vi "Main.vi"() -> ()   [LabVIEW 2011]
uses:
  2-Think/2 Typedefs/Which Boat.ctl
  2-Think/2 Typedefs/UTM Circle.ctl
  0x2-OCU-Think Comm/0x2 Typedefs/Waypoints List.ctl
  2-Think/2 Classes/Waypoint/Waypoint.lvclass
  0x2-OCU-Think Comm/0x2 Typedefs/Current Waypoint.ctl
  2-Think/2 Typedefs/eStopCommand.ctl
  0x2-OCU-Think Comm/0x2 Typedefs/ocuMessage.ctl
  0x2-OCU-Think Comm/0x2 Typedefs/ocuCommands.ctl
  <vilib>/Platform/TimedLoop/XDataNode/timing_clust.ctl
  <vilib>/Platform/TimedLoop/XDataNode/nitl_modes.ctl
  <vilib>/Platform/TimedLoop/XDataNode/wakeup.ctl
  <vilib>/vision/Image Controls.llb/IMAQ Image.ctl
  2-Think/2 Globals/2 Global.vi
  2-Think/2 Globals/2 Message Logger.vi
  <vilib>/Platform/TimedLoop/XDataNode/XDataNode.xnode
  <vilib>/Platform/TimedLoop/XDataNode/XDNodeRunTimeDep.lvlib
  0x2-OCU-Think Comm/0x2 Classes/NetworkStreams/Writer/NetworkStreamWriter.lvclass
  0x2-OCU-Think Comm/0x2 Classes/NetworkStreams/Reader/NetworkStreamReader.lvclass
  2-Think/2 Classes/Logger/Logger.lvclass
panel:
  in  "Skip Sense (->manual input only!)":bool
  in  "Enable logging?":bool=TRUE
  in  "Data storage folder":path
  in  "Which Boat Am I?\n(unnecessary to set on RIO)":T1=enum."Simulation"
  out "E-stop freq.":dbl
  out "Act freq.":dbl
  out "Sense freq.":dbl
  out "Think freq.":dbl
  in  "E-Stop":bool
  # "this is the parent VI under which \nSense Think and Act run."
  # "Will save to U:\\Logs when run on the RIO"
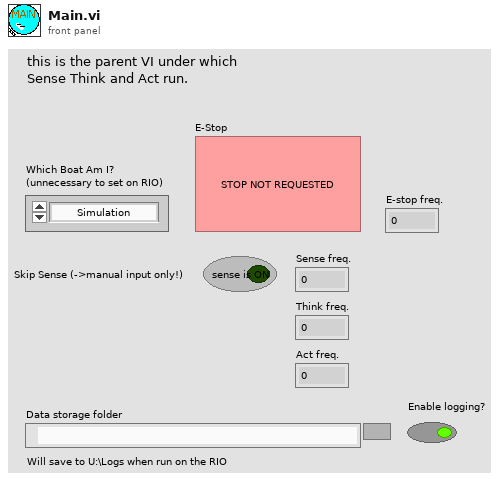
[diagram p1: front panel]
types:
  T1 = typedef "Which Boat.ctl" = enum16{"Competition Boat", "Small RC", "Simulation"}
  T2 = typedef "UTM Circle.ctl" = cluster{"UTM Zone":dbl, "Hemisphere":enum16{"North", "South"}, "East":dbl, "North":dbl, "Radius":dbl}
  T3 = typedef "Waypoints List.ctl" = refnum<class "Waypoint.lvclass">[]
  T4 = typedef "Current Waypoint.ctl" = i32
  T5 = typedef "eStopCommand.ctl" = enum16{"Reset E-Stop", "Get E-Stop", "Set E-Stop"}
  T6 = typedef "ocuMessage.ctl" = cluster{"OCU Command":T7, "Data":variant}
  T7 = typedef "ocuCommands.ctl" = enum16{"Pass", "Send override", "Add waypoint", "Delete waypoint", "Set waypoint number", "Stop", "Add Mission", "Reset Missions/Waypts", "Edit Control Values", "Add Global No-Sail", "Log Message"}
  T8 = typedef "XDNodeRunTimeDep.lvlib/timing_clust.ctl" = cluster{"Expected End [f-1]":u64, "Actual End [f-1]":u64, "Finished Late? [f-1]":bool, "Expected End [i-1]":u64, "Actual End [i-1]":u64, "Finished Late? [i-1]":bool, "Expected Start [i]":u64, "Actual Start [i]":u64, "Expected Start [f]":u64, "Actual Start [f]":u64, "Source Name":string, "Structure Name":string, "Period":i64, "Deadline":i64, "Offset":i64, "Start":i64, "Priority":i32, "Timeout":i32, "Mode":T9, "Wakeup Reason":T10, "Error":errorcluster, "Source Type":string, "Secondary Source Type":string, "Global End Time":u64, "Global Start Time":u64, "Frame Duration":u64, "Iteration Duration":u64, "Assigned CPU":i32, "I/O Scan Engine Mode":u32}
  T9 = typedef "XDNodeRunTimeDep.lvlib/nitl_modes.ctl" = enum32{"No Change", "Process missed periods, maintain original phase", "Discard missed periods, maintain original phase", "Process missed periods, ignore original phase", "Discard missed periods, ignore original phase"}
  T10 = typedef "XDNodeRunTimeDep.lvlib/wakeup.ctl" = enum32{"Normal", "Aborted", "Asynchronous wakeup", "Timing source error", "Timed loop error", "Timeout"}
  T11 = typedef "IMAQ Image.ctl" = refnum<image>
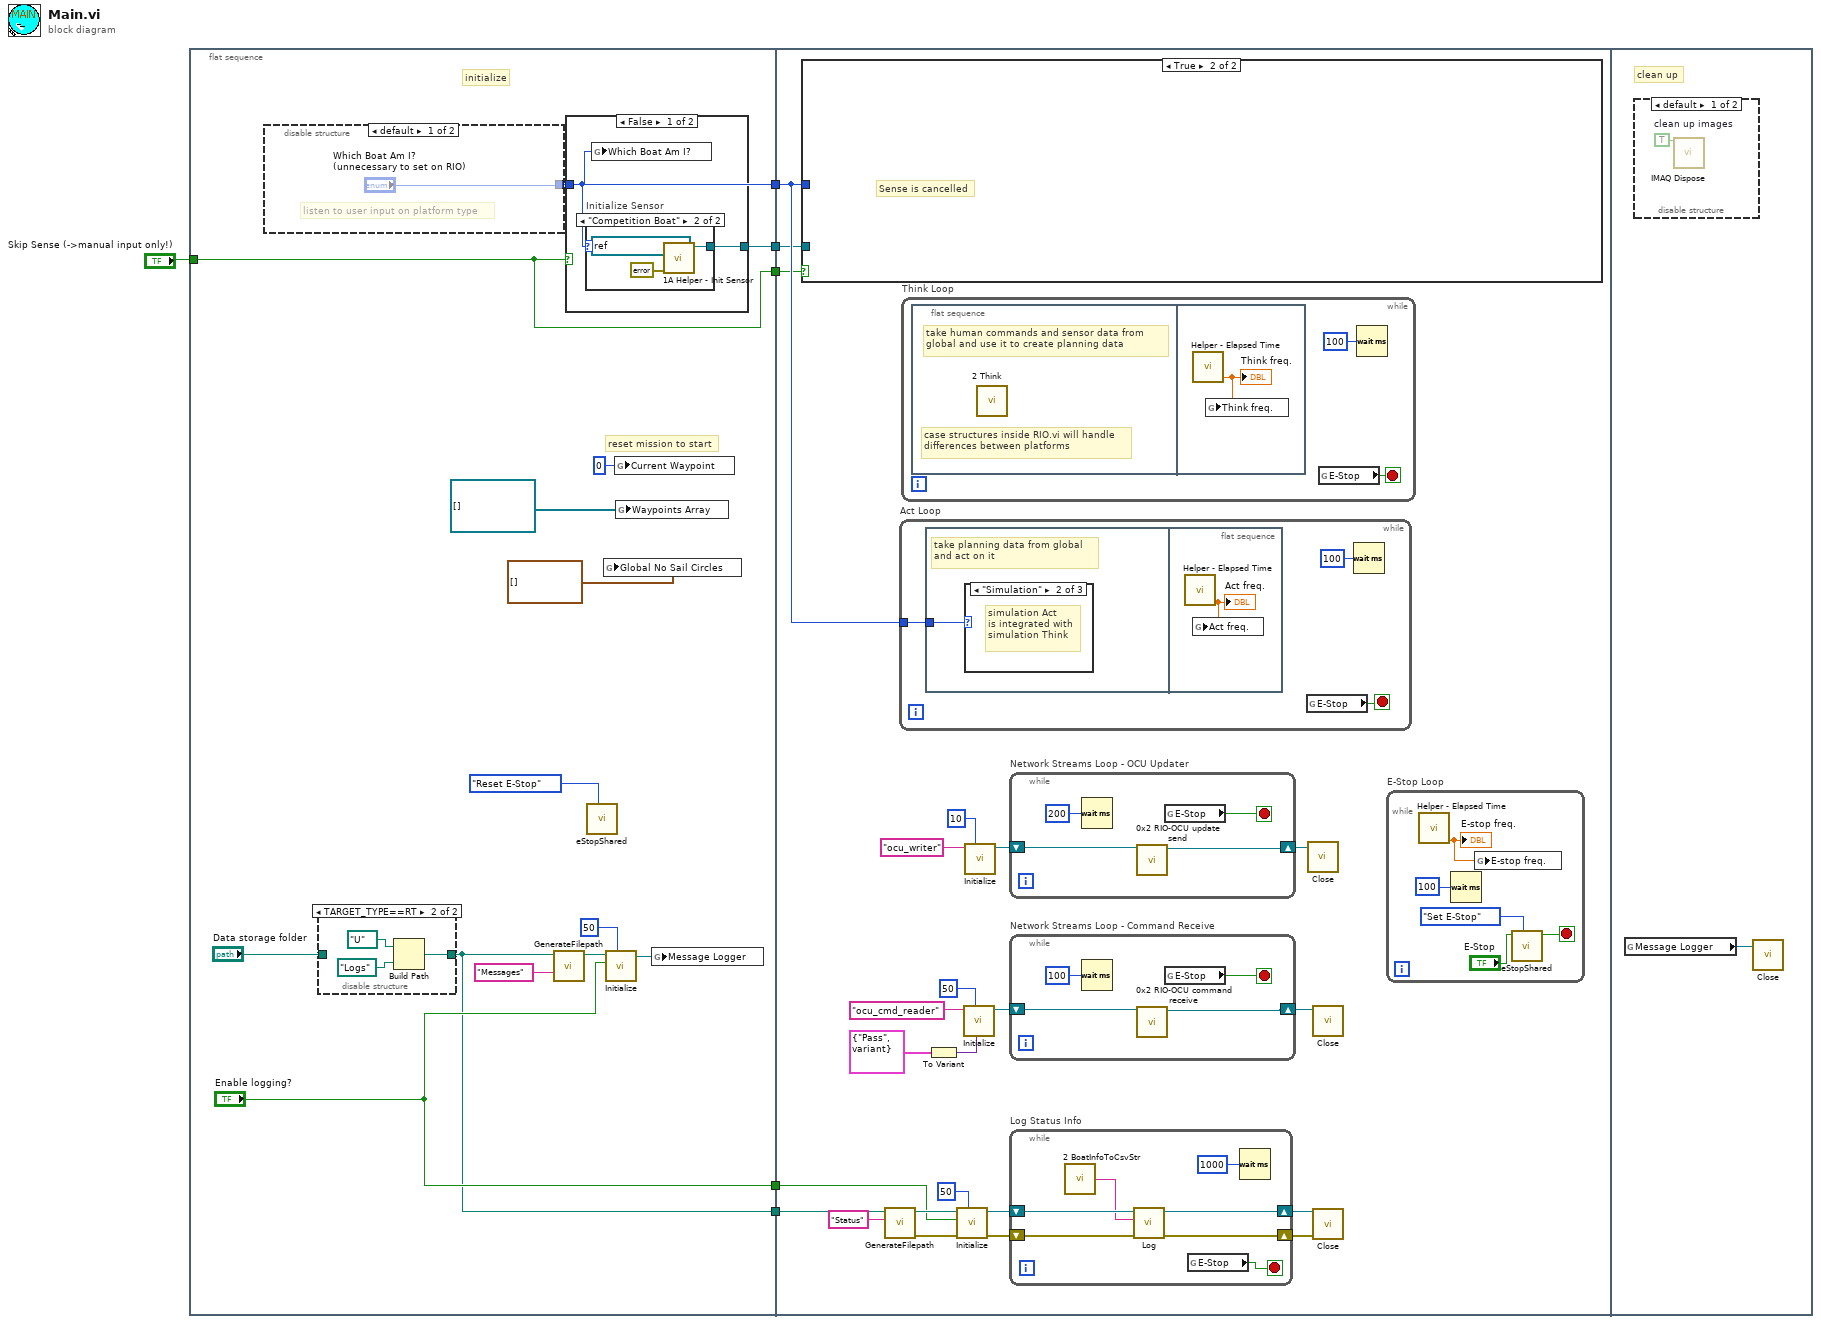
[diagram p0: block diagram]
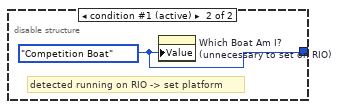
[diagram p5: hidden frame]
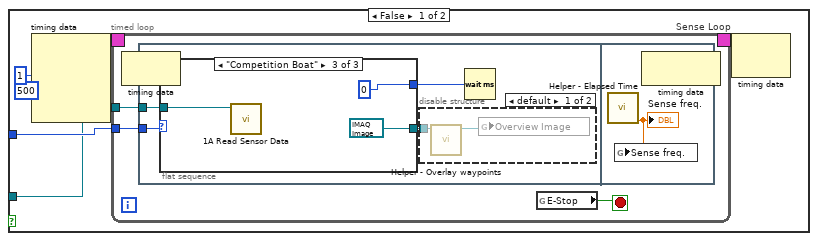
[diagram p6: hidden frame]
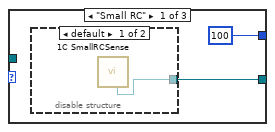
[diagram p8: hidden frame]
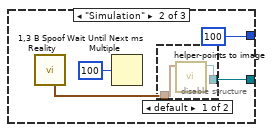
[diagram p10: hidden frame]
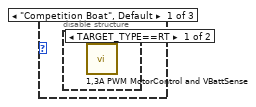
[diagram p12: hidden frame]
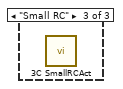
[diagram p14: hidden frame]
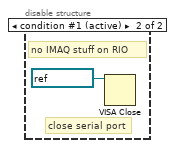
[diagram p15: hidden frame]
diagram:
  n1 = flat-sequence {
    tunnel: [w17] -> w6
    tunnel: [w18] -> w5
    tunnel: [w10] -> w4
    tunnel: ["Enable logging?"] -> w3
    tunnel: "Skip Sense (->manual input only!)" -> [w8]
    tunnel: [w8] -> w1
    tunnel: w6 -> [w54]
    tunnel: w5 -> [w53]
    tunnel: w4 -> [w37]
    tunnel: w3 -> [w33]
    tunnel: w1 -> [w32]
    frame #0 {
      # "reset mission to start"
      # "initialize"
      n2 = disable-structure shown="default" {
        disable-tunnel: ["Which Boat Am I?\n(unnecessary to set on RIO)" w31] -> w17
        frame condition #0 {
          # "listen to user input on platform type"
        }
        frame condition #1 (active) {
          w31 = Which_Boat."Competition Boat" ("Which Boat Am I?")
          # "detected running on RIO -> set platform"
          n3 = property on="Which Boat Am I?\n(unnecessary to set on RIO)" class="Enum (strict)"("Value"=w31) -> ()  [unwired: 2 in, 2 out]
        }
      }
      n4 = disable-structure shown="TARGET_TYPE==RT" {
        disable-tunnel: "Data storage folder" -> [w26 _]
        disable-tunnel: [w26 w27] -> w10
        frame condition #0 {
        }
        frame condition #1 (active) {
          n5 = Build Path(base path=path "U:/" ("Data storage folder"), name or relative path=path "Logs" ("Data storage folder")) -> (appended path=w27:path)
        }
      }
      n6 = call "GenerateFilepath.vi"("Identifier"="Messages", "Data storage folder"=w10) -> ("File path out"=w13:path)  [unwired: 8 in, 1 out]
      n7 = case shown="False" w8 {
        tunnel: [w22 _] -> w18
        tunnel: w17 -> [w21 _]
        frame False {
          n8 = case "Initialize Sensor" shown="\"Competition Boat\"" w21 {
            tunnel: [_ w23] -> w22
            frame Default {
            }
            frame "Competition Boat" {
              n9 = call "1A Helper - Init Sensor.vi"("error in (no error)"=errorcluster {"status"=FALSE, "code"=0, "source"=""}, "VISA Refnum in"=refnum<visa-resource-name> "ASRL1::INSTR" ("VISA resource name")) -> ("VISA Refnum out"=w23:refnum<visa-resource-name>)  [unwired: 7 in, 2 out]
            }
          }
          n10 = global write "2 Global.vi" "Which Boat Am I?"(w21) -> ()
        }
        frame True {
        }
      }
      n11 = call "eStopShared.vi"("Command"=eStopCommand."Reset E-Stop") -> ()  [unwired: 9 in, 2 out]
      n12 = global write "2 Global.vi" "Global No Sail Circles"(T2[] [] ("Global No Sail Circles")) -> ()
      n13 = call "Initialize.vi"("buffer size"=50, "Enable? (T)"="Enable logging?", "File path"=w13) -> ("Logger out"=w14:refnum<class "Logger.lvclass">)  [unwired: 7 in, 1 out]
      n14 = global write "2 Global.vi" "Current Waypoint"(T4 0 ("Current Waypoint")) -> ()
      n15 = global write "2 Global.vi" "Waypoints Array"(T3 [] ("Waypoints Array")) -> ()
      n16 = global write "2 Message Logger.vi" "Message Logger"(w14) -> ()
    }
    frame #1 {
      n17 = case shown="True" w32 {
        tunnel: w54 -> [w58 _]
        tunnel: w53 -> [w57 _]
        frame False {
          n18 = node-c288(i64 1 ("Period"), 500 ("Priority")) -> (w60:T8)  [unwired: 2 in]
          n19 = timed-loop "Sense Loop" {
            tunnel: w58 -> [w62]
            tunnel: w57 -> [w61]
            timing: w60 -> [_]
            timing-out: [_] -> w59
            stop <- w63 stop-if-true
            n20 = node-c288() -> ()  [unwired: 1 in, 1 out]
            n21 = flat-sequence {
              tunnel: w62 -> [w68]
              tunnel: w61 -> [w66]
              frame #0 {
                n22 = case shown="\"Competition Boat\"" w68 {
                  tunnel: [w73 w76 T11 refnum ("Image Out")] -> w69
                  tunnel: [u32 100 ("millisecond multiple") u32 100 ("millisecond multiple") u32 0 ("millisecond multiple")] -> w67
                  tunnel: w66 -> [_ _ w81]
                  frame "Small RC" {
                    n23 = disable-structure shown="default" {
                      disable-tunnel: [w74 _] -> w73
                      frame condition #0 {
                        n24 = call "1C SmallRCSense.vi"() -> ("Eye in the Sky"=w74:T11)  [unwired: 6 in, 5 out]
                      }
                      frame condition #1 (active) {
                      }
                    }
                  }
                  frame "Simulation" {
                    n25 = call "1,3 B Spoof Reality.vi"() -> ("Boat Path"=w77:cluster{"X Position":dbl, "Y Position":dbl}[])  [unwired: 5 in, 6 out]
                    n26 = Wait Until Next ms Multiple(millisecond multiple=u32 100) -> ()  [unwired: 1 out]
                    n27 = disable-structure shown="default" {
                      disable-tunnel: w77 -> [w80 _]
                      disable-tunnel: [w79 _] -> w76
                      frame condition #0 {
                        n28 = call "helper-points to image.vi"("Array of Points"=w80) -> ("Image Out"=w79:T11)  [unwired: 10 in]
                      }
                      frame condition #1 (active) {
                        # "no IMAQ\non RIO"
                      }
                    }
                  }
                  frame "Competition Boat" {
                    n29 = call "1A Read Sensor Data.vi"("VISA resource name (in)"=w81) -> ()  [unwired: 9 in, 2 out]
                  }
                }
                n30 = disable-structure shown="default" {
                  disable-tunnel: w69 -> [w70 _]
                  frame condition #0 {
                    n31 = call "Helper - Overlay waypoints.vi"("Img Refnum in"=w70) -> ("Img Refnum out"=w71:T11)  [unwired: 10 in]
                    n32 = global write "2 Global.vi" "Overview Image"(w71) -> ()
                  }
                  frame condition #1 (active) {
                    # "no IMAQ stuff on RIO"
                  }
                }
                n33 = Wait (ms)(milliseconds to wait=w67) -> ()  [unwired: 1 out]
              }
              frame #1 {
                n34 = call "Helper - Elapsed Time.vi"() -> ("Frequency (Hz)"=w84:dbl)  [unwired: 10 in, 1 out]
                "Sense freq." <- w84
                n35 = global write "2 Global.vi" "Sense freq."(w84) -> ()
              }
            }
            n36 = global read "2 Global.vi" "E-Stop"() -> (w63:bool)
            n37 = node-c288() -> ()  [unwired: 1 in, 1 out]
          }
          n38 = node-c288(w59) -> ()  [unwired: 1 out]
        }
        frame True {
          # "Sense is cancelled"
        }
      }
      n39 = call "GenerateFilepath.vi"("Identifier"="Status", "Data storage folder"=w37) -> ("error out"=w41:errorcluster, "File path out"=w42:path)  [unwired: 8 in]
      n40 = while "Act Loop" {
        tunnel: w54 -> [w114]
        stop <- w115 stop-if-true
        n41 = flat-sequence {
          tunnel: w114 -> [w116]
          frame #0 {
            # "take planning data from global\nand act on it"
            n42 = case shown="\"Simulation\"" w116 {
              frame "Competition Boat", Default {
                n43 = disable-structure shown="TARGET_TYPE==RT" {
                  frame condition #0 (active) {
                    n44 = call "1,3A PWM MotorControl and VBattSense.vi"() -> ()  [unwired: 12 in]
                  }
                  frame condition #1 {
                  }
                }
              }
              frame "Simulation" {
                # "simulation Act\nis integrated with\nsimulation Think"
              }
              frame "Small RC" {
                n45 = call "3C SmallRCAct.vi"() -> ()  [unwired: 12 in]
              }
            }
          }
          frame #1 {
            n46 = call "Helper - Elapsed Time.vi"() -> ("Frequency (Hz)"=w117:dbl)  [unwired: 10 in, 1 out]
            "Act freq." <- w117
            n47 = global write "2 Global.vi" "Act freq."(w117) -> ()
          }
        }
        n48 = global read "2 Global.vi" "E-Stop"() -> (w115:bool)
        n49 = Wait (ms)(milliseconds to wait=u32 100 ("millisecond multiple")) -> ()  [unwired: 1 out]
      }
      n50 = while "Think Loop" {
        stop <- w111 stop-if-true
        n51 = flat-sequence {
          frame #0 {
            # "case structures inside RIO.vi will handle\ndifferences between platforms"
            # "take human commands and sensor data from\nglobal and use it to create planning data"
            n52 = call "2 Think.vi"() -> ()  [unwired: 12 in]
          }
          frame #1 {
            n53 = call "Helper - Elapsed Time.vi"() -> ("Frequency (Hz)"=w112:dbl)  [unwired: 10 in, 1 out]
            "Think freq." <- w112
            n54 = global write "2 Global.vi" "Think freq."(w112) -> ()
          }
        }
        n55 = global read "2 Global.vi" "E-Stop"() -> (w111:bool)
        n56 = Wait (ms)(milliseconds to wait=u32 100 ("millisecond multiple")) -> ()  [unwired: 1 out]
      }
      n57 = To Variant(anything=T6 {"OCU Command"=enum."Pass", "Data"=variant} ("OCU Message")) -> (Variant=w48:variant)
      n58 = call "Initialize.vi"("buffer size"=50, "error in (no error)"=w41, "Enable? (T)"=w33, "File path"=w42) -> ("error out"=w38:errorcluster, "Logger out"=w39:refnum<class "Logger.lvclass">)  [unwired: 6 in]
      n59 = call "Initialize.vi"("Default return"=w48, "reader buffer size"=50 ("writer buffer size"), "reader name"="ocu_cmd_reader") -> ("NetworkStreamWriter out"=w44:refnum<class "NetworkStreamReader.lvclass">)  [unwired: 6 in, 2 out]
      n60 = call "Initialize.vi"("writer buffer size"=10, "writer name"="ocu_writer") -> ("NetworkStreamWriter out"=w52:refnum<class "NetworkStreamWriter.lvclass">)  [unwired: 7 in, 2 out]
      n61 = while "Network Streams Loop - OCU Updater" {
        shift-right: [w101] -> w51
        shift-left: w52 -> [w102]
        stop <- w104 stop-if-true
        n62 = Wait (ms)(milliseconds to wait=u32 200 ("millisecond multiple")) -> ()  [unwired: 1 out]
        n63 = call "0x2 RIO-OCU update send.vi"("OCU Writer In"=w102) -> ("OCU Writer Out"=w101:refnum<class "NetworkStreamWriter.lvclass">)  [unwired: 10 in]
        n64 = global read "2 Global.vi" "E-Stop"() -> (w104:bool)
      }
      n65 = while "Network Streams Loop - Command Receive" {
        shift-right: [w97] -> w45
        shift-left: w44 -> [w98]
        stop <- w100 stop-if-true
        n66 = Wait (ms)(milliseconds to wait=u32 100 ("millisecond multiple")) -> ()  [unwired: 1 out]
        n67 = call "0x2 RIO-OCU command receive.vi"("Manual Override Reader In"=w98) -> ("Manual Override Reader Out"=w97:refnum<class "NetworkStreamReader.lvclass">)  [unwired: 10 in]
        n68 = global read "2 Global.vi" "E-Stop"() -> (w100:bool)
      }
      n69 = while "Log Status Info" {
        shift-right: [w94] -> w35
        shift-left: w39 -> [w95]
        shift-right: [w93] -> w34
        shift-left: w38 -> [w92]
        stop <- w96 stop-if-true
        n70 = call "2 BoatInfoToCsvStr.vi"() -> ("Log String"=w90:string)  [unwired: 1 in]
        n71 = call "Log.vi"("error in (no error)"=w92, "Message"=w90, "Logger in"=w95) -> ("error out"=w93:errorcluster, "Logger out"=w94:refnum<class "Logger.lvclass">)  [unwired: 7 in]
        n72 = global read "2 Global.vi" "E-Stop"() -> (w96:bool)
        n73 = Wait (ms)(milliseconds to wait=u32 1000 ("millisecond multiple")) -> ()  [unwired: 1 out]
      }
      n74 = call "Close.vi"("NetworkStreamWriter in"=w51) -> ()  [unwired: 9 in, 2 out]
      n75 = call "Close.vi"("NetworkStreamReader in"=w45) -> ()  [unwired: 9 in, 2 out]
      n76 = call "Close.vi"("error in (no error)"=w34, "NetworkStreamWriter in"=w35) -> ()  [unwired: 9 in, 1 out]
      n77 = while "E-Stop Loop" {
        stop <- w106 stop-if-true
        n78 = call "Helper - Elapsed Time.vi"() -> ("Frequency (Hz)"=w105:dbl)  [unwired: 10 in, 1 out]
        "E-stop freq." <- w105
        n79 = Wait (ms)(milliseconds to wait=u32 100 ("millisecond multiple")) -> ()  [unwired: 1 out]
        n80 = global write "2 Global.vi" "E-stop freq."(w105) -> ()
        n81 = call "eStopShared.vi"("Command"=eStopCommand."Set E-Stop", "E-Stop"="E-Stop") -> ("E-Stop Out"=w106:bool)  [unwired: 8 in, 1 out]
      }
    }
    frame #2 {
      # "clean up"
      n82 = global read "2 Message Logger.vi" "Message Logger"() -> (w118:refnum<class "Logger.lvclass">)
      n83 = disable-structure shown="default" {
        frame condition #0 {
          w119 = TRUE  # clean up images
          n84 = call "IMAQ Dispose"("All Images? (No)"=w119) -> ()  [unwired: 5 in, 1 out]
        }
        frame condition #1 (active) {
          # "close serial port"
          # "no IMAQ stuff on RIO"
          n85 = VISA Close(VISA resource name=refnum<visa-resource-name> "COM1") -> ()  [unwired: 1 in, 1 out]
        }
      }
      n86 = call "Close.vi"("NetworkStreamWriter in"=w118) -> ()  [unwired: 10 in, 1 out]
    }
  }
